vi "Unibot.vi"() -> ()   [LabVIEW 2012]
doc: "Pendubot (Pendulum Robot) consists of a DC motor connected to a link physical rigid link (called here 'elbow\") which is connected to a second rigid link ('arm\") that has no actuation (free spinning link).\n\nThe control objective is to keep the free link in the vertical position while you can choose to balance the controller link (called here elbow) in the extended position (both links are up) or in the contracted position (elbow pointing down and free link up). In those operating points, a State Feedback Control is used to keep in Up-Up or Down-Up position.\n\nThis VI demonstrates how to use Linearization, design of LQR and pole placement controllers and use on swiching controller."
uses:
  <vilib>/addons/Control Design/_Model Construction/Model Typedefs.llb/CD State Space Model (MIMO).ctl
  <vilib>/addons/Control Design/_Model Construction/Model Typedefs.llb/CD General Elements.ctl
  <vilib>/Simulation/Scripting/Companion Diagram/SimConfigNode/SimParams.ctl
  <vilib>/Simulation/Scripting/Companion Diagram/SimConfigNode/_simSolvers.ctl
  <vilib>/Simulation/Implementation/Shared/SIMSCR Execution Mode.ctl
  <vilib>/Platform/TimedLoop/XDataNode/timing_clust.ctl
  <vilib>/Platform/TimedLoop/XDataNode/nitl_modes.ctl
  <vilib>/Platform/TimedLoop/XDataNode/wakeup.ctl
  <vilib>/Simulation/Param Hierarchy/Typedefs/SIMPH Param Control Actions.ctl
  <vilib>/Simulation/Scripting/Editor Utilities/SIM subVI tag data.ctl
  <vilib>/Simulation/Scripting/Editor Utilities/SIM subVI execution type.ctl
  <vilib>/Simulation/Implementation/Shared/NILVSim_ParamChanged.vi
  <vilib>/Simulation/Implementation/Shared/NILVSim_FinishedLate.vi
  <vilib>/Simulation/Utility/Implementation/SIM Halt.vi
  <vilib>/Simulation/SignalDisplay/Implementation/NILVSim Time Waveform.llb/SIM Time Waveform (scalar).vi
  <vilib>/Simulation/Implementation/Shared/SIM Fire Discrete SubVI.vi
  <vilib>/Simulation/Implementation/Shared/NILVSim_Manager.vi
  <vilib>/Simulation/Implementation/Shared/NILVSim_FinalizeModel.vi
  <vilib>/Simulation/Utility/Implementation/NILVSim Memory.llb/NILVSim Memory (core).vi
  <vilib>/Simulation/Implementation/Shared/SIM Fire Discrete SubVI (Core).vi
  <vilib>/addons/Control Design/_State Feedback Control/State Feedback Control.llb/State Feedback Control SubVis/cd_Discretized Linear Quadratic Regulator.vi
  <vilib>/Simulation/Implementation/Shared/SIM Unbundle Sim Info.vi
  <vilib>/Utility/error.llb/Clear Errors.vi
  <vilib>/Simulation/Implementation/Shared/NILVSim_GetModelError.vi
  <vilib>/Simulation/Implementation/Shared/SIM Bundle Sim Info.vi
  <vilib>/Simulation/Implementation/Shared/SIMSH Read Queue.vi
  <vilib>/Simulation/Implementation/Shared/NILVSim_Initialize.vi
  <vilib>/Simulation/Utility/Implementation/NILVSim Get Time and IsAcceptedStep.vi
  <vilib>/addons/Control Design/_Utility/Model Viewer.llb/Model Viewer SubVI/cd_Draw State-Space Equation (SS).vi
  <vilib>/addons/Control Design/_Model Conversions/Continuous and Discrete.llb/Continuous and Discrete SubVI/cd_Convert Continuous to Discrete (SS).vi
  <vilib>/addons/Control Design/_State Feedback Control/State Feedback Control.llb/CD State Regulator.vi
  <vilib>/addons/Control Design/_Model Reduction/Model Reduction.llb/Model Reduction SubVIs/cd_Remove I-O-S from SS Model.vi
  <vilib>/addons/Control Design/_Dynamic Analysis/Dynamic Analysis.llb/Dynamic Analysis subVI/cd_Stability (State-Space).vi
  <vilib>/addons/Control Design/_Dynamic Analysis/Dynamic Analysis.llb/Dynamic Analysis subVI/cd_Pole-Zero Map (State-Space).vi
  <vilib>/addons/Control Design/_Frequency Response Analysis/Frequency Response.llb/Frequency Response subVI/cd_Bode (State Space).vi
  <vilib>/addons/Control Design/_Time Response Analysis/Time Response.llb/Time Response subVI/cd_Impulse Response (State-Space).vi
  <vilib>/addons/Control Design/_Time Response Analysis/Time Response.llb/Time Response subVI/cd_Parametric Time Response (SS with External Response).vi
  Unibot - State Machine Controller.vi
  <vilib>/Simulation/Scripting/Companion Diagram/SimConfigNode/SimDog.xnode
  UniPend - NonLinear Model.vi
  <vilib>/Platform/TimedLoop/XDataNode/XDataNode.xnode
  <vilib>/Simulation/Implementation/XNodeFramework/SimXNode/SimX.xnode
  Unibot - Nonlinear Model.vi
  <vilib>/addons/Control Design/_State Feedback Control/NI_CD_State Feedback Control.lvlib
  <vilib>/addons/Control Design/_Utility/NI_CD_Model Viewer.lvlib
  <vilib>/addons/Control Design/_Model Reduction/NI_CD_Model Reduction.lvlib
  <vilib>/addons/Control Design/_Time Response Analysis/NI_CD_Time Response.lvlib
  <vilib>/addons/Control Design/_Utility/NI_LinSys_Polynomial Math.lvlib
  <vilib>/addons/Control Design/_Frequency Response Analysis/NI_CD_Frequency Response.lvlib
  <vilib>/addons/Control Design/_Model Conversions/NI_CD_Continuous and Discrete.lvlib
  <vilib>/addons/Control Design/_Dynamic Analysis/NI_CD_Dynamic Analysis.lvlib
  <vilib>/Platform/TimedLoop/XDataNode/XDNodeRunTimeDep.lvlib
  <vilib>/Simulation/Implementation/Shared/NI_SIM_Implementation.lvlib
  <vilib>/addons/Control Design/_Model Construction/NI_LinSys_Model Typedefs.lvlib
panel:
  out "Gain":dbl[][](array[numeric])=[[13.362365480735772, 19.05380394095224, 1.2104119144158012, 2.4013527998190582]]
  out "State-Space Model":T1={"properties"={"Model name"="", "Input names"=["Torque (Tau)"], "Output names"=["theta1", "theta2"], "Input Delays"=[0.0], "Output Delays"=[0.0, 0.0], "Sampling Time"=0.0, "Notes"=""}, "A"=[[0.0, 0.0, 1.0, 0.0], [0.0, 0.0, 0.0, 1.0], [-54.92473360770753, 40.408778283769514, -1.4920114239882594, 7.105427357601002e-15], [45.63201235945519, 58.19855210917706, 1.492011423988302, -0.22573956409963358]], "B"=[[0.0], [0.0], [29.84022847976503], [3.9334375679108007]], "C"=[[1.0, 0.0, 0.0, 0.0], [0.0, 0.9999999998433566, 0.0, 0.0]], "D"=[[0.0], [0.0]], "StateNames"=["/teta1", "/teta2", "/dteta1", "/dteta2"], "Transport Delay"=[[0.0], [0.0]]} {"Transport Delay" format="%.2f"; "D" format="%#.2g"; "C" format="%#.2g"; "B" format="%#.2g"; "A" format="%#.2g"; "properties"."Sampling Time" format="%#.6p"; "properties"."Output Delays" format="%.4f"; "properties"."Input Delays" format="%.4f"}
  in  "PD Gains":T3={"Kp Up"=16.55, "Kd Up"=5.1567, "Kp Down"=10.2, "Kd Down"=0.974}
  in  "Tab Control":T4(tab)
  in  "Start Open Loop":bool
  out "torque 2":waveform(dbl)(graph)={"t0"=timestamp(0 s since 1904-01-01), "dt"=1.0, "Y"=[0.0]}
  out "3D Picture Control 2":refnum<vi>(3d-picture)
  out "teta1 2":waveform(dbl)(graph)={"t0"=timestamp(0 s since 1904-01-01), "dt"=1.0, "Y"=[0.0]}
  in  "Initial Alpha (Angle)":dbl(knob) scale=-3.14..3.14
  in  "Iitial Beta":dbl(knob) scale=-3.14..3.14
  in  "Right":bool
  in  "Intensity":dbl(slide)=10.0 scale=0.0..10.0
  in  "Left":bool
  in  "Control Technique":T5(tab)
  in  "Q":dbl[][](array[numeric])=[[10.0, 0.0], [0.0, 10.0]] format="%.2f"
  in  "R":dbl[][](array[numeric])=[[50.0]] format="%.2f"
  in  "Desired Pole Location":cdb[](array[numeric])=[0.8275428216771237+0.0i, 0.9068860314786581+0.0i, 0.9511525717602396+0.0i, 0.9425028249515996+0.0i] format="%.2f"
  out "Optimal Gain \nDown-Up":dbl[](array[numeric])=[13.362365480735772, 19.05380394095224, 1.2104119144158012, 2.4013527998190582] format="%.2f"
  out "Optimal Gain\nDown-Down":dbl[](array[numeric])=[-0.14906178101626644, 0.17686358569380023, 1.1761652926773682, -0.039275718443801] format="%.2f"
  out "Optimal Gain \nUp-Up":dbl[](array[numeric])=[-16.081278889113918, -16.397482495141958, -3.1902773104017657, -2.0364914176335533] format="%.2f"
  in  "Type of Control":bool=TRUE
  out "Linearized Equation for Operating Point":picture
  out "Poles locations":cdb[](array[numeric])=[0.6612119646152013+0.0i, 0.9743397418352502+0.0i, 0.9379855295915182+0.0i, 0.9275584671894643+0.0i] format="%.2f"
  out "Impulse Response":cluster{"time":dbl[], dbl[]}[](graph)
  out "Settling Time 1":dbl=2.363776391897807
  out "Settling Time 2":dbl=2.488531257025747
  out "Bode Magnitude":cluster{"W":dbl[], "Magnitude":dbl[]}[](graph)
  out "Bode Phase":cluster{"W":dbl[], "Magnitude":dbl[]}[](graph)
  out "Pole-Zero Map":cluster{dbl[], dbl[]}[](graph)=[{[-30.459733943866535, -2.5043848732190277, -7.159085784207853, -7.159085784207853], [0.0, 0.0, 0.6196593444828095, -0.6196593444828095]}, {[], []}] caption="Closed Loop System Poles"
  out "Stability":T6(ring)
  out "Zeros":cdb[](array[numeric]) format="%.4f"
  out "Poles":cdb[](array[numeric])=[-30.459733943866535+0.0i, -2.5043848732190277+0.0i, -7.159085784207853+0.6196593444828095i, -7.159085784207853-0.6196593444828095i] format="%.4f"
  out "3D Picture Control":refnum<vi>(3d-picture)
  out "teta1":waveform(dbl)(graph)={"t0"=timestamp(0 s since 1904-01-01), "dt"=1.0, "Y"=[12.566370614359172]}
  out "teta2":waveform(dbl)(graph)={"t0"=timestamp(0 s since 1904-01-01), "dt"=1.0, "Y"=[0.0]}
  out "torque":waveform(dbl)(graph)={"t0"=timestamp(0 s since 1904-01-01), "dt"=1.0, "Y"=[0.0]}
  in  "Halt?":bool
  in  "Kill?":bool
  out "Switching State":string="Bringing home"
  in  "Setpoint":dbl(knob) step=0.01 scale=-0.1..0.1
  in  "Enable?":bool
  in  "Control":bool=TRUE
  # "Pendubot - two link Pendulum with \"elbow\" control"
  # "Objective:"
  # "Pendubot (Pendulum Robot) consists of a DC motor connected to a link physical rigid link (called here 'elbow\") which is connected to a second rigid link ('arm\") that has no actuation (free spinning link).\nThe control objective is to keep the free link in the vertical position while you can choose to balance the controller link (called here elbow) in the extended position (both links are up) or in the contracted position (elbow pointing down and free link up). In those operating points, a State Feedback Control is used to keep in Up-Up or Down-Up position. You can tune those controllers in the Design Tab. The controller also can switch between Down-Down position to any other using state machine to apply another control laws to get to the desired location. The technique used for this operation is called partial feedback linearization and PD controllers were used to implement this system. This example also uses a state-machine to switch between states. To avoid chaotic fall of the pendulum if it can't reach the position, another controller is used to drive the elbow to the stationary position (elbow and free link pointing down)."
  # "Variables:\nTorque (Tau): Voltage applied controller\nTheta1: Encoder Position of the controlled link*\nTheta2: Encoder Position of the free link*\n\n*Enconders have zero reference point down"
  # "Up-Up Position"
  # "Down-Down Position"
  # "Down-Up Position"
  # "In this position, the\nelbow is pointing down and free link is controlled in the up position."
  # "In this position, the elbow and free link are pointing down. This is also a stable position and simulation starts from this point."
  # "In this position, the\nelbow and free link is controlled in the up position, similar to an inverted pendulum."
  # "Disturbance"
  # "Description:"
  # "The allow the system of such complex machine, we need to develop control techniques based on different states. We have a total of 7 controllers that are controlled by a state-macine that switches whenever the condition is stabilished. The \"down-down\"position is considered to be initial state. Whenever the system doesn't meet specific command, the state machine will bring the system to the down-down position. This controller is designed using a Linear Quadratic Regulator with the model linearized at the down-down position. \n\nTo transition between the Down-Down position to Down-Up and Up-Up position, it is used a nonlinear control technique called \"Feedback Linearization\". The implementation of the controller is using a Proportional-Derivative (PD) controller, which is tuned by 'experimentation' in this case.\n\nThe same LQR technique is applied to obtain the controller around the Up-Up and the Down-Up position.  The gain are designed in the 'Control Design' tab and your objective is to choose the gain that makes the controller stable and resistent to disturbance."
  # "State Feedback Controller\nwith state machine"
  # "Initialize"
  # "Swing Up?"
  # "Swing Down?"
  # "Down-Down\nPosition"
  # "Feedback\nlinearization\nPD controller"
  # "Feedback\nlinearization\nPD controller"
  # "Out of\n bounds?"
  # "Out of\n bounds?"
  # "State\nFeedback\nDown-Down"
  # "In bounds?"
  # "In bounds?"
  # "State\nFeedback\nDown-Up"
  # "State\nFeedback\nUp-Up"
  # "Home?"
  # "Home?"
  # "Encoder\nMeasurements\n(Theta1 and Theta 2)"
  # "DC Motor"
  # "State Feedback Controller\nwith state machine"
  # "Swing Up?"
  # "Swing Down?"
  # "Initialize"
  # "Home?"
  # "Home?"
  # "Control Technique"
  # "Desired\nOperating\nPoint"
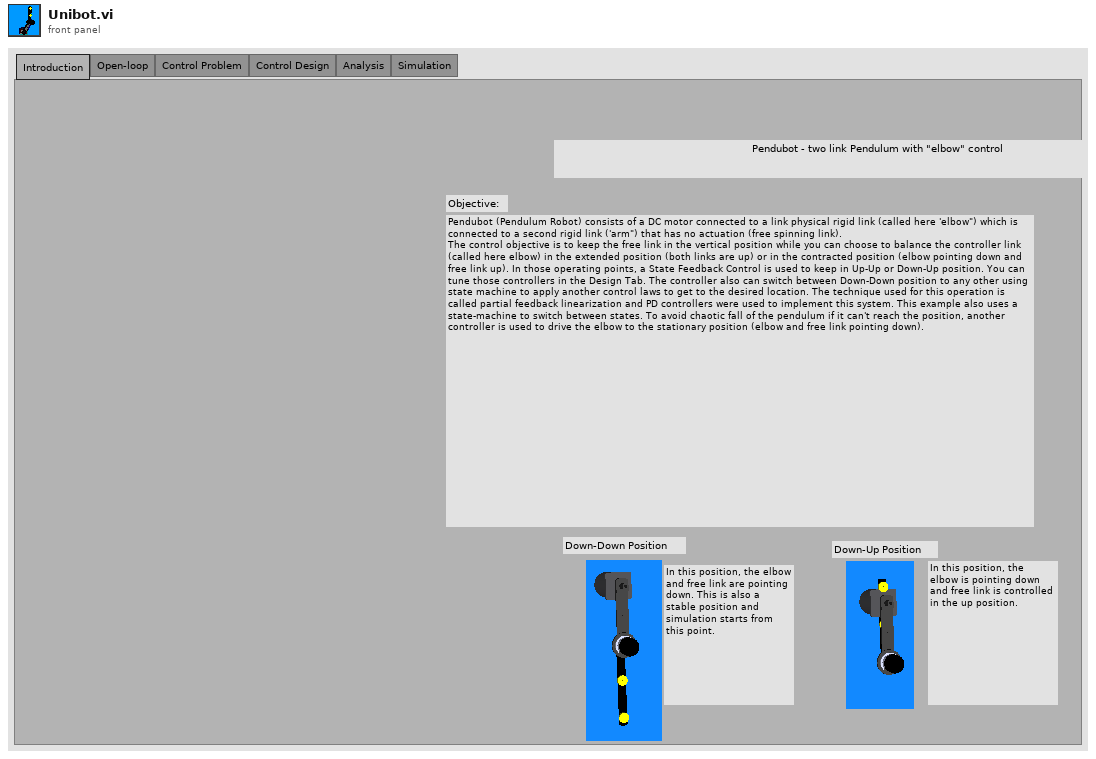
[diagram p1: front panel]
types:
  T1 = typedef "NI_LinSys_Model Typedefs.lvlib/CD State Space Model (MIMO).ctl" = cluster{"properties":T2, "A":dbl[][], "B":dbl[][], "C":dbl[][], "D":dbl[][], "StateNames":string[], "Transport Delay":dbl[][]}
  T2 = typedef "NI_LinSys_Model Typedefs.lvlib/CD General Elements.ctl" = cluster{"Model name":string, "Input names":string[], "Output names":string[], "Input Delays":dbl[], "Output Delays":dbl[], "Sampling Time":dbl, "Notes":string}
  T3 = cluster{"Kp Up":dbl, "Kd Up":dbl, "Kp Down":dbl, "Kd Down":dbl}
  T4 = enum32{"Introduction", "Open-loop", "Control Problem", "Control Design", "Analysis", "Simulation"}
  T5 = enum32{"Linear Quadratic Regulator", "Pole Placement"}
  T6 = enum16{"stable", "marginally stable", "unstable", "undetermined"}
  T7 = typedef "SIMSCR Execution Mode.ctl" = enum16{"Simulate to Completion", "Single Time-Step Simulation (Fixed Step Only)"}
  T8 = typedef "XDNodeRunTimeDep.lvlib/timing_clust.ctl" = cluster{"Expected End [f-1]":u64, "Actual End [f-1]":u64, "Finished Late? [f-1]":bool, "Expected End [i-1]":u64, "Actual End [i-1]":u64, "Finished Late? [i-1]":bool, "Expected Start [i]":u64, "Actual Start [i]":u64, "Expected Start [f]":u64, "Actual Start [f]":u64, "Source Name":string, "Structure Name":string, "Period":i64, "Deadline":i64, "Offset":i64, "Start":i64, "Priority":i32, "Timeout":i32, "Mode":T9, "Wakeup Reason":T10, "Error":errorcluster, "Source Type":string, "Secondary Source Type":string, "Global End Time":u64, "Global Start Time":u64, "Frame Duration":u64, "Iteration Duration":u64, "Assigned CPU":i32, "I/O Scan Engine Mode":u32}
  T9 = typedef "XDNodeRunTimeDep.lvlib/nitl_modes.ctl" = enum32{"No Change", "Process missed periods, maintain original phase", "Discard missed periods, maintain original phase", "Process missed periods, ignore original phase", "Discard missed periods, ignore original phase"}
  T10 = typedef "XDNodeRunTimeDep.lvlib/wakeup.ctl" = enum32{"Normal", "Aborted", "Asynchronous wakeup", "Timing source error", "Timed loop error", "Timeout"}
  T11 = typedef "SIMPH Param Control Actions.ctl" = enum16{"get params", "set params"}
  T12 = typedef "SIM subVI tag data.ctl" = cluster{"period":dbl, "skew":dbl, "Simulation execution type":T13}
  T13 = typedef "SIM subVI execution type.ctl" = enum16{"Function call", "Discrete", "Continuous", "Initialization only", "Final step only"}
  T14 = cluster{"SIMSH Sim Time":dbl, "Build Array":cluster{"appended array":dbl[]}, "Unwrap Phase PtByPt.vi":cluster{"unwrapped phase":dbl}, "dalpha":cluster{"output":dbl}, "alpha":cluster{"output":dbl}, "Add 6":cluster{"x+y":dbl}, "Subtract 2":cluster{"x-y":dbl}, "Add 5":cluster{"x+y":dbl}, "Quotient & Remainder 2":cluster{"x-y*floor(x/y)":dbl}, "Multiply 8":cluster{"x*y":dbl}, "Formula Node":cluster{"d2alpha":dbl}}
  T15 = typedef "SimParams.ctl" = cluster{"Initial Time (s)":dbl, "Final Time (s)":dbl, "Step Size (s)":dbl, "ODE Solver":T16, "Minimum Step Size (s)":dbl, "Maximum Step Size (s)":dbl, "Relative Tolerance":dbl, "Absolute Tolerance":dbl, "Software Timing":bool, "Initial Step Size (s)":dbl, "Automatic Fixed Step Size?":bool, "Automatic Discrete Step Size?":bool, "Discrete Step Size (s)":dbl, "Calculate using Time Step":bool, "Solver Wired?":bool, "Prev.Frm.Expected End":u64, "Prev.Frm.Actual End":u64, "Prev.Frm.Finished Late?":bool, "Prev.Iter.Expected End":u64, "Prev.Iter.Actual End":u64, "Prev.Iter.Finished Late?":bool, "Expected Iteration Start":u64, "Actual Iteration Start":u64, "Expected Frame Start":u64, "Actual Frame Start":u64, "Source Name":string, "Name":string, "Period":i64, "Deadline":i64, "Offset":i64, "Start":i64, "Priority":i32, "Timeout":i32, "Processor":i32, "Mode":enum32{"No Change", "Process missed periods, maintain original phase", "Discard missed periods, maintain original phase", "Process missed periods, ignore original phase", "Discard missed periods, ignore original phase"}, "Wakeup reason":enum32{"Normal", "Aborted", "Asynchronous wakeup", "Timing source error", "Timed loop error", "Timeout"}, "Error":errorcluster, "Source Type":string, "Secondary Source Type":string, "Global End Time":u64, "Global Start Time":u64, "Full Solver Reset":bool, "Execution Mode":T7, "Nan/Inf Check":bool, "Custom Solver Library":string, "Solver Is Variable":bool, "custom solver name":string, "Signal Collection Decimation":u32}
  T16 = typedef "_simSolvers.ctl" = enum16{"Runge-Kutta 1 (Euler)", "Runge-Kutta 2", "Runge-Kutta 3", "Runge-Kutta 4", "Runge-Kutta 23 (variable)", "Runge-Kutta 45 (variable)", "BDF (variable)", "Adams-Moulton (variable)", "Rosenbrock (variable)", "Discrete States Only", "SDIRK 4 (variable)", "Radau 5 (variable)", "Radau 9 (variable)", "Radau 13 (variable)", "Radau [Variable Order] (variable)", "Gear's Method (variable)", "Linearizer", "State Query", "Trim Eval", "Custom Solver"}
  T17 = enum16{"System Included", "System Included with Noise", "Standalone"}
  T18 = cluster{"SIMSH Sim Time":dbl, "Unwrap Phase PtByPt.vi 2":cluster{"unwrapped phase":dbl}, "Unwrap Phase PtByPt.vi":cluster{"unwrapped phase":dbl}, "dteta1":cluster{"output":dbl}, "teta1":cluster{"output":dbl}, "dteta2":cluster{"output":dbl}, "teta2":cluster{"output":dbl}, "Add 6":cluster{"x+y":dbl}, "Subtract 2":cluster{"x-y":dbl}, "Add 5":cluster{"x+y":dbl}, "Quotient & Remainder 2":cluster{"x-y*floor(x/y)":dbl}, "Subtract":cluster{"x-y":dbl}, "Add 4":cluster{"x+y":dbl}, "Constant":dbl, "Quotient & Remainder":cluster{"x-y*floor(x/y)":dbl}, "Multiply 8":cluster{"x*y":dbl}, "Build Array":cluster{"appended array":dbl[]}, "Formula Node":cluster{"d2teta1":dbl, "d2teta2o":dbl}, "Add 3":cluster{"x+y":dbl}, "Multiply 7":cluster{"x*y":dbl}, "Square 2":cluster{"x^2":dbl}, "Multiply 6":cluster{"x*y":dbl}, "Compound Arithmetic":cluster{"result":dbl}, "Multiply 5":cluster{"x*y":dbl}, "Add 2":cluster{"x+y":dbl}, "Multiply 4":cluster{"x*y":dbl}, "Multiply 3":cluster{"x*y":dbl}, "Multiply 2":cluster{"x*y":dbl}, "Multiply":cluster{"x*y":dbl}, "Add":cluster{"x+y":dbl}, "Square":cluster{"x^2":dbl}}
  T19 = enum8{"Enabled", "Disabled", "Disabled and Grayed Out"}
  T20 = typedef "NI_LinSys_Data Typedefs.lvlib/CD MIMO Time Response Data.ctl" = cluster{"Time":dbl[], "Outputs Data":dbl[][][], "States Data":dbl[][][], "plot type":T21}
  T21 = typedef "NI_LinSys_Data Typedefs.lvlib/CD Plot Types Enum.ctl" = enum16{"bode-magnitude", "bode-phase", "nichols", "nyquist", "singular values", "step", "impulse", "initial", "simulation", "nyquist with separation"}
  T22 = typedef "NI_LinSys_Data Typedefs.lvlib/CD Parametric Time Response Data.ctl" = cluster{"Rise Time (s)":dbl[][], "Peak Time (s)":dbl[][], "Settling Time (s)":dbl[][], "Overshoot (%)":dbl[][], "Steady-State Gain":dbl[][], "Peak Value":dbl[][]}
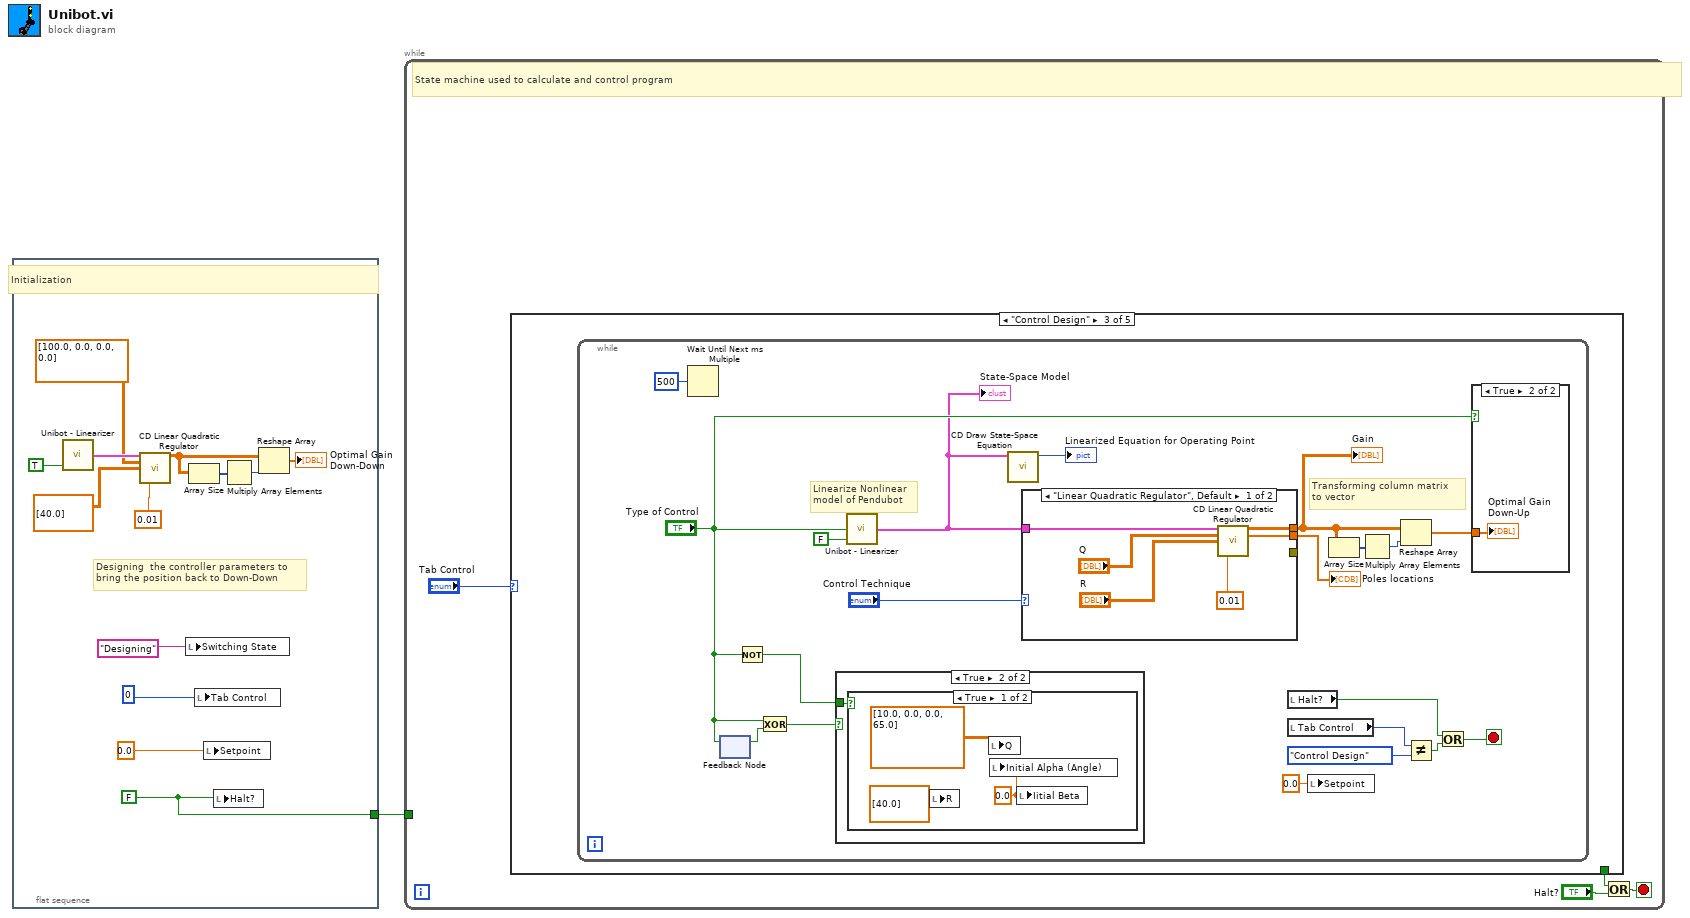
[diagram p0: block diagram]
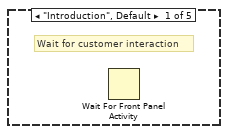
[diagram p2: hidden frame]
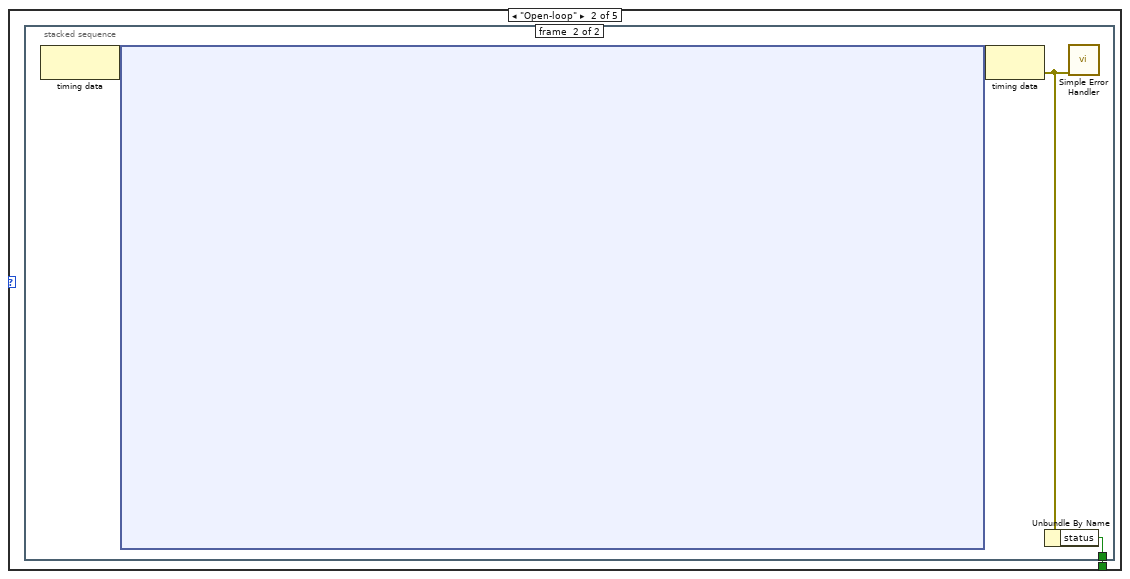
[diagram p3: hidden frame]
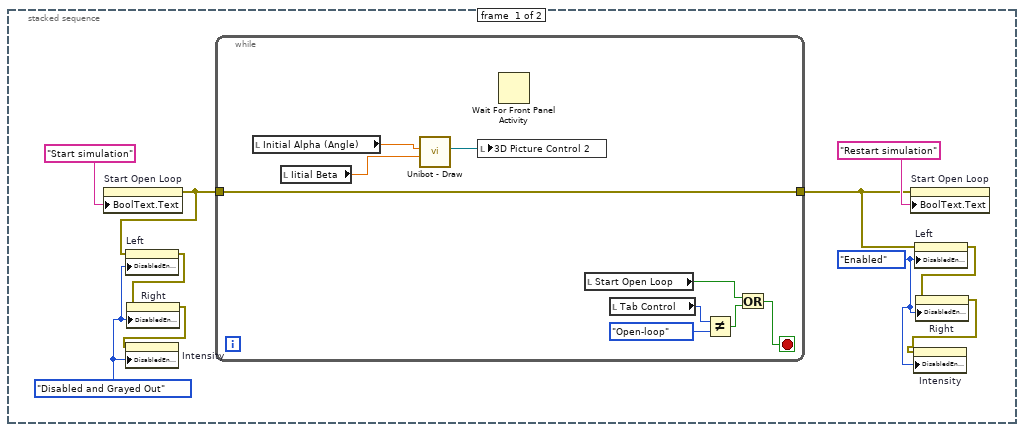
[diagram p4: hidden frame]
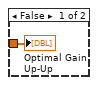
[diagram p5: hidden frame]
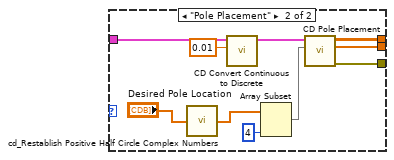
[diagram p6: hidden frame]
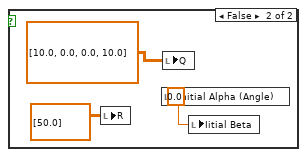
[diagram p8: hidden frame]
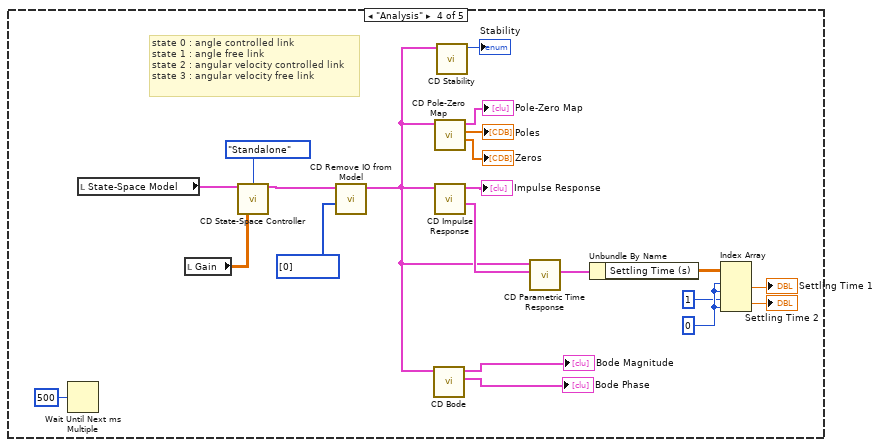
[diagram p9: hidden frame]
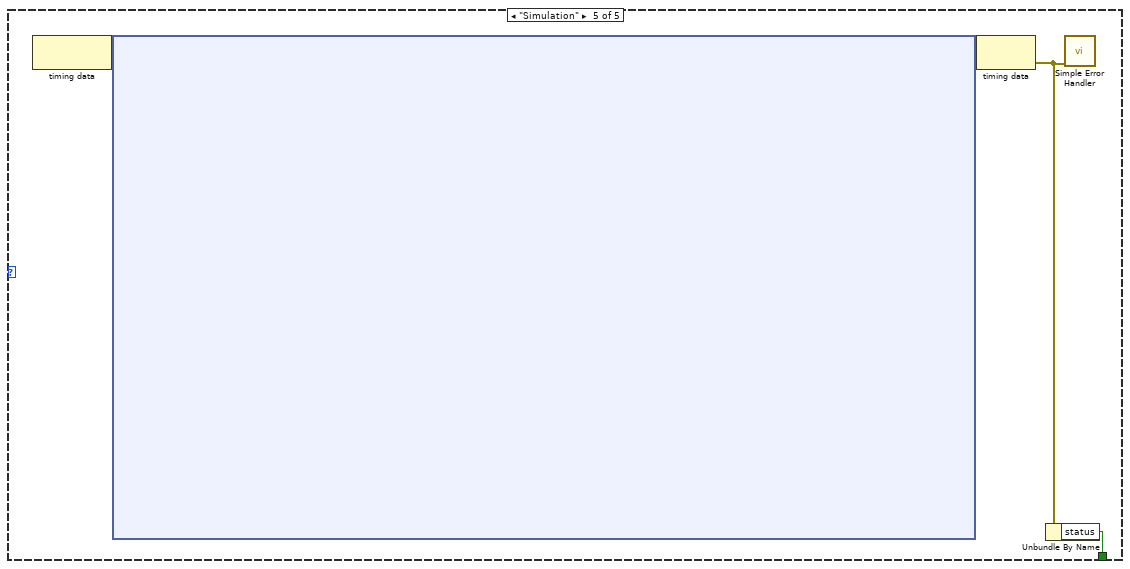
[diagram p10: hidden frame]
diagram:
  n1 = flat-sequence {
    tunnel: [w13] -> w1
    frame #0 {
      w13 = FALSE ("Halt?")
      # "Designing  the controller parameters to \nbring the position back to Down-Down"
      # "Initialization"
      n2 = call "Unibot - Linearizer.vi"("Up-Up"=TRUE ("Down-Down")) -> ("State-Space Model"=w11:T1)  [unwired: 1 in, 3 out]
      n3 = call-poly <vilib>:"CD Linear Quadratic Regulator.vi"("Continuous State-Space Model"=w11, "Q"=dbl[][] [[100.0, 0.0], [0.0, 0.0]], "R"=dbl[][] [[40.0]], "Sampling Time (s)"=0.01) -> ("Optimal Gain (K)"=w8:dbl[][])  [unwired: 2 in, 9 out]
      n4 = local write "Switching State"("Designing" ("Switching State")) -> ()
      n5 = Array Size(array=w8) -> (size(s)=w10:i32[])
      n6 = local write "Tab Control"(0 ("Setpoint")) -> ()
      n7 = local write "Setpoint"(0.0 ("Setpoint")) -> ()
      n8 = local write "Halt?"(w13) -> ()
      n9 = Multiply Array Elements(1:w10) -> (0:w9:i32)
      n10 = Reshape Array(w8, w9) -> (→"Optimal Gain\nDown-Down":dbl[])
    }
  }
  n11 = while {
    tunnel: w1 -> [_]
    stop <- w16 stop-if-true
    # "State machine used to calculate and control program"
    n12 = case shown="\"Control Design\"" "Tab Control" {
      tunnel: [_ w19 _ _ w478] -> w15
      frame "Introduction", Default {
        # "Wait for customer interaction"
        n13 = Wait For Front Panel Activity() -> ()  [unwired: 3 in, 1 out]
      }
      frame "Open-loop" {
        n14 = stacked-sequence {
          tunnel: [_ w39] -> w19
          frame #0 {
            w23 = T19."Disabled and Grayed Out" ("Disabled")
            w20 = T19."Enabled" ("Disabled")
            n15 = property on="Start Open Loop" class="Bool (strict)"("BoolText.Text"="Start simulation" ("Boolean Text.Text")) -> (error out=w26:errorcluster)  [unwired: 2 in, 1 out]
            n16 = property on="Left" class="Bool (strict)"(error in=w26, "DisabledEnum"=w23) -> (error out=w24:errorcluster)  [unwired: 1 in, 1 out]
            n17 = property on="Right" class="Bool (strict)"(error in=w24, "DisabledEnum"=w23) -> (error out=w22:errorcluster)  [unwired: 1 in, 1 out]
            n18 = property on="Intensity" class="Slide (strict)"(error in=w22, "DisabledEnum"=w23) -> ()  [unwired: 1 in, 2 out]
            n19 = while {
              tunnel: w26 -> [w30]
              tunnel: [w30] -> w27
              stop <- w31 stop-if-true
              n20 = local read "Initial Alpha (Angle)"() -> (w37:dbl)
              n21 = local read "Iitial Beta"() -> (w36:dbl)
              n22 = call "Unibot - Draw.vi"("Frame"=w36, "Motor"=w37) -> ("Rotated Scene Object"=w38:refnum<vi>)  [unwired: 9 in]
              n23 = local write "3D Picture Control 2"(w38) -> ()
              n24 = Wait For Front Panel Activity() -> ()  [unwired: 3 in, 1 out]
              n25 = local read "Start Open Loop"() -> (w32:bool)
              n26 = local read "Tab Control"() -> (w35:T4)
              n27 = Not Equal?(x=w35, y=T4."Open-loop") -> (x != y?=w33:bool)
              n28 = Or(x=w32, y=w33) -> (x .or. y?=w31:bool)
            }
            n29 = property on="Start Open Loop" class="Bool (strict)"(error in=w27, "BoolText.Text"="Restart simulation" ("Boolean Text.Text")) -> ()  [unwired: 1 in, 2 out]
            n30 = property on="Left" class="Bool (strict)"(error in=w27, "DisabledEnum"=w20) -> (error out=w25:errorcluster)  [unwired: 1 in, 1 out]
            n31 = property on="Right" class="Bool (strict)"(error in=w25, "DisabledEnum"=w20) -> (error out=w21:errorcluster)  [unwired: 1 in, 1 out]
            n32 = property on="Intensity" class="Slide (strict)"(error in=w21, "DisabledEnum"=w20) -> ()  [unwired: 1 in, 2 out]
          }
          frame #1 {
            n33 = node-c288() -> (w42:variant)  [unwired: 1 out]
            n34 = node-c254 ("Simulation Loop")(w42) -> (w41:variant)
            n35 = node-c288(w41) -> (w40:errorcluster)
            n36 = Unbundle By Name(w40) -> ("status"=w39:bool)
            n37 = call <vilib>:"Simple Error Handler.vi"("error in (no error)"=w40) -> ()  [unwired: 1 in, 8 out]
          }
        }
      }
      frame "Control Design" {
        n38 = while {
          stop <- w421 stop-if-true
          # "Linearize Nonlinear\nmodel of Pendubot"
          # "Transforming column matrix\nto vector"
          n39 = Wait Until Next ms Multiple(millisecond multiple=u32 500) -> ()  [unwired: 1 out]
          n40 = feedback-in #1("Type of Control") -> ()
          n41 = feedback #1() -> (w427:bool)  [unwired: 1 out]
          n42 = Not(x="Type of Control") -> (.not. x?=w425:bool)
          n43 = Exclusive Or(1:w427, 2:"Type of Control") -> (0:w426:bool)
          n44 = case shown="True" w426 {
            tunnel: w425 -> [_ w448]
            frame False {
            }
            frame True {
              n45 = case shown="True" w448 {
                frame True {
                  w449 = 0.0 ("initial teta2")
                  n46 = local write "R"(dbl[][] [[40.0]] ("R")) -> ()
                  n47 = local write "Q"(dbl[][] [[10.0, 0.0], [0.0, 65.0]] ("Q")) -> ()
                  n48 = local write "Initial Alpha (Angle)"(w449) -> ()
                  n49 = local write "Iitial Beta"(w449) -> ()
                }
                frame False {
                  w452 = 0.0 ("initial teta1")
                  n50 = local write "R"(dbl[][] [[50.0]] ("R")) -> ()
                  n51 = local write "Initial Alpha (Angle)"(w452) -> ()
                  n52 = local write "Q"(dbl[][] [[10.0, 0.0], [0.0, 10.0]] ("Q")) -> ()
                  n53 = local write "Iitial Beta"(w452) -> ()
                }
              }
            }
          }
          n54 = call "Unibot - Linearizer.vi"("Type of Control"="Type of Control", "Up-Up"=FALSE ("Down-Down")) -> ("State-Space Model"=w412:T1)  [unwired: 3 out]
          "State-Space Model" <- w412
          n55 = call-poly <vilib>:"CD Draw State-Space Equation.vi"("State-Space Model"=w412) -> ("Equation"=→"Linearized Equation for Operating Point":picture)  [unwired: 4 in, 6 out]
          n56 = case shown="\"Linear Quadratic Regulator\", Default" "Control Technique" {
            tunnel: [w437 w447] -> w413
            tunnel: w412 -> [w436 w443]
            tunnel: [w433 w446] -> w419
            tunnel: [_ w444] -> _
            frame "Linear Quadratic Regulator", Default {
              n57 = call-poly <vilib>:"CD Linear Quadratic Regulator.vi"("Continuous State-Space Model"=w436, "Q"="Q", "R"="R", "Sampling Time (s)"=0.01) -> ("Optimal Gain (K)"=w437:dbl[][], "Eigenvalues"=w433:cdb[])  [unwired: 2 in, 8 out]
            }
            frame "Pole Placement" {
              n58 = call <vilib>:"cd_Restablish Positive Half Circle Complex Numbers.vi"("Sorted Complex Numbers (Positive Only)"="Desired Pole Location") -> ("Complete Roots"=w440:cdb[])  [unwired: 8 out]
              n59 = call-poly <vilib>:"CD Convert Continuous to Discrete.vi"("Sampling Time (s)"=0.01, "Continuous State-Space Model"=w443) -> ("Discrete State-Space Model"=w442:T1)  [unwired: 7 in, 2 out]
              n60 = Array Subset(array=w440, length=4) -> (w438:cdb[])  [unwired: 1 in]
              n61 = call <vilib>:"CD Pole Placement.vi"("Poles"=w438, "State-Space Model"=w442) -> ("error out"=w444:errorcluster, "Actual Poles"=w446:cdb[], "Gain"=w447:dbl[][])  [unwired: 2 in, 5 out]
            }
          }
          "Poles locations" <- w419
          "Gain" <- w413
          n62 = local read "Halt?"() -> (w422:bool)
          n63 = local read "Tab Control"() -> (w420:T4)
          n64 = local write "Setpoint"(0.0 ("Gauge")) -> ()
          n65 = Array Size(array=w413) -> (size(s)=w429:i32[])
          n66 = Multiply Array Elements(1:w429) -> (0:w428:i32)
          n67 = Reshape Array(w413, w428) -> (w417:dbl[])
          n68 = Not Equal?(x=w420, y=T4."Control Design") -> (x != y?=w423:bool)
          n69 = Or(x=w422, y=w423) -> (x .or. y?=w421:bool)
          n70 = case shown="True" "Type of Control" {
            tunnel: w417 -> [w430 w431]
            frame False {
              "Optimal Gain \nUp-Up" <- w430
            }
            frame True {
              "Optimal Gain \nDown-Up" <- w431
            }
          }
        }
      }
      frame "Analysis" {
        w466 = 0 ("index (row)")
        # "state 0 : angle controlled link\nstate 1 : angle free link\nstate 2 : angular velocity controlled link\nstate 3 : angular velocity free link"
        n71 = Wait Until Next ms Multiple(millisecond multiple=u32 500) -> ()  [unwired: 1 out]
        n72 = local read "State-Space Model"() -> (w474:T1)
        n73 = local read "Gain"() -> (w472:dbl[][])
        n74 = call-poly <vilib>:"CD State-Space Controller.vi"("State-Space Model"=w474, "Configuration"=T17."Standalone", "Controller Gain (K)"=w472) -> ("Controller Model"=w471:T1)  [unwired: 11 in, 1 out]
        n75 = call-poly <vilib>:"CD Remove IO from Model.vi"("State-Space Model"=w471, "Outputs"=i32[] [0]) -> ("Reduced Model"=w459:T1)  [unwired: 7 in, 1 out]
        n76 = call-poly <vilib>:"CD Bode.vi"("State-Space Model"=w459) -> ("Bode Phase"=→"Bode Phase":cluster{"W":dbl[], "Magnitude":dbl[]}[], "Bode Magnitude"=→"Bode Magnitude":cluster{"W":dbl[], "Magnitude":dbl[]}[])  [unwired: 6 in, 3 out]
        n77 = call-poly <vilib>:"CD Pole-Zero Map.vi"("State-Space Model"=w459) -> ("Zeros"=→"Zeros":cdb[], "Poles"=→"Poles":cdb[], "Pole-Zero Map"=→"Pole-Zero Map":cluster{dbl[], dbl[]}[])  [unwired: 7 in, 1 out]
        n78 = call-poly <vilib>:"CD Impulse Response.vi"("State-Space Model"=w459) -> ("Impulse Response Data"=w469:T20, "Impulse Response Graph"=→"Impulse Response":cluster{"time":dbl[], dbl[]}[])  [unwired: 7 in, 2 out]
        n79 = call-poly <vilib>:"CD Stability.vi"("State-Space Model"=w459) -> ("Stability"=→"Stability":T6)  [unwired: 8 in, 2 out]
        n80 = call-poly <vilib>:"CD Parametric Time Response.vi"("Time Response Data"=w469, "State-Space Model"=w459) -> ("Time Response Parametric Data"=w468:T22)  [unwired: 8 in, 1 out]
        n81 = Unbundle By Name(w468) -> ("Settling Time (s)"=w460:dbl[][])
        n82 = Index Array(array=w460, index (row) #1=w466, index (col) #1=w466, index (row) #2=1 ("index (row)"), index (col) #2=w466) -> (element #1=→"Settling Time 1":dbl, element #2=→"Settling Time 2":dbl)
      }
      frame "Simulation" {
        n83 = node-c288() -> (w477:variant)  [unwired: 1 out]
        n84 = node-c254 ("Simulation Loop 2")(w477) -> (w476:variant)
        n85 = node-c288(w476) -> (w479:errorcluster)
        n86 = Unbundle By Name(w479) -> ("status"=w478:bool)
        n87 = call <vilib>:"Simple Error Handler.vi"("error in (no error)"=w479) -> ()  [unwired: 1 in, 8 out]
      }
    }
    n88 = Or(x=w15, y="Halt?") -> (x .or. y?=w16:bool)
  }
